vi "RTM Add Calculations.vi"(8 "error in (no error)":errorcluster, 11 "Node Ptr":u64 format="%.0x") -> (0 "error out":errorcluster)   [LabVIEW 2015, in "Waveform-Processing-Custom-Device System Explorer.lvlib"]
uses:
  Waveform-Processing-Custom-Device System Explorer.lvlib
  NationalInstruments.VeriStand.SystemStorageUI
  Classes/RunningAverageCalculation/RunningAverageCalculation.lvclass
  Classes/ScaledWaveformCalculation/ScaledWaveformCalculation.lvclass
  Classes/LatestValueCalculation/LatestValueCalculation.lvclass
  Shared/Constants.vi
  <vilib>/NI Veristand/Custom Device API/Get Item Property (String Array).vi
  NationalInstruments.VeriStand.SystemStorage
  Classes/WaveformCalculation/WaveformCalculation.lvclass
  <vilib>/NI VeriStand/Custom Device API/Custom Device API.lvlib
  <vilib>/NI VeriStand/UI Controls/System Definition Tree/NI_VS UI System Tree.lvlib
  Shared/Waveform-Processing-Custom-Device Shared.lvlib
  <vilib>/NI VeriStand/Custom Device Tools/Custom Device Utility Library/Custom Device Utility Library.lvlib
panel:
  in  "Select a calculation:":u16(ring)
  in  "OK Button":bool
  in  "TreeBrowserWF":refnum<k24>(container)
  in  "Tag":string
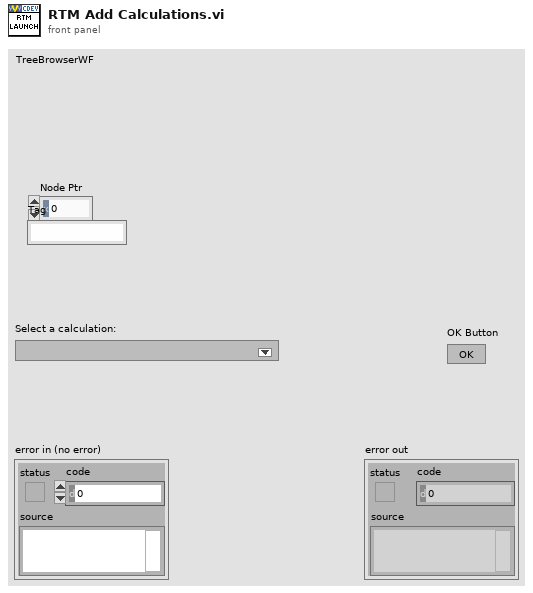
[diagram p1: front panel]
types:
  T1 = typedef "Custom Device API.lvlib/Custom Device Item Ref.ctl" = u64
  T2 = typedef "Custom Device API.lvlib/Custom Device Pointer.ctl" = refnum<k24>
  T3 = typedef "NI_VS UI System Tree.lvlib/Callback Type.ctl" = cluster{"Net Callbacks":refnum<k27>[], "Event":T4}
  T4 = typedef "NI_VS UI System Tree.lvlib/Net Event Data Ref.ctl" = refnum<user-event>
  T5 = typedef "NI_VS UI System Tree.lvlib/System Definition Tree Ref.ctl" = refnum<k24>
  T6 = typedef "Custom Device API.lvlib/Custom Device Item Info.ctl" = cluster{"Name":string, "Is Channel":bool, "GUID":string, "Is Waveform":bool}
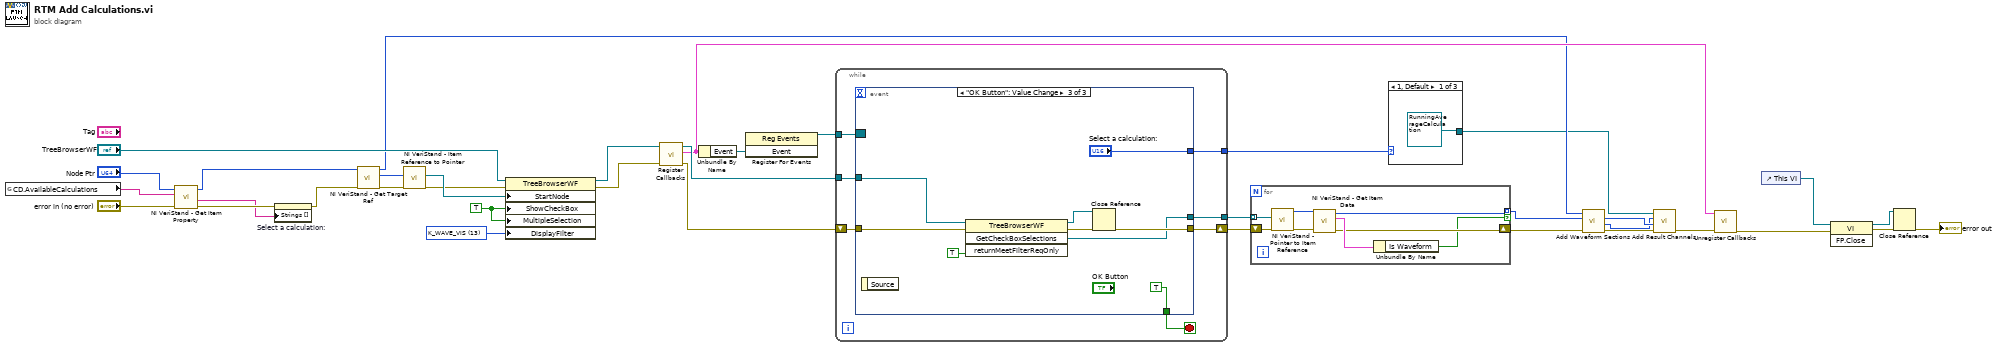
[diagram p0: block diagram]
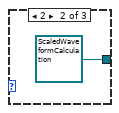
[diagram p2: hidden frame]
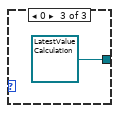
[diagram p3: hidden frame]
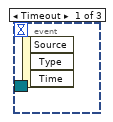
[diagram p4: hidden frame]
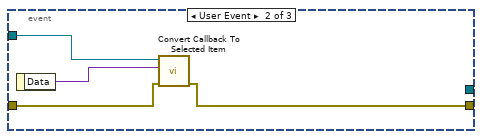
[diagram p5: hidden frame]
diagram:
  w24 = u8 13 items=["K_CHAN_R", "K_CHAN_W", "K_CHAN_RW", "K_CHAN_VOLT", "K_CHAN_FAULT", "K_ALL", "K_CUSTOM", "K_CHAN_R_VIS", "K_CHAN_W_VIS", "K_CHAN_RW_VIS", "K_CHAN_VOLT_VIS", "K_CHAN_FAULT_VIS", "K_WAVE", "K_WAVE_VIS", "K_WAVE_DBL", "K_WAVE_CDB", "K_WAVE_DBL_VIS", "K_WAVE_CDB_VIS"] ("filterType")
  w30 = TRUE ("ShowCheckBox")
  n1 = global read "Constants.vi" "CD.AvailableCalculations"() -> (w19:string)
  n2 = call-poly <vilib>:"NI VeriStand - Get Item Property.vi"("error in (no error)"="error in (no error)", "Property Name"=w19, "Item Ref in"="Node Ptr") -> ("error out"=w20:errorcluster, "Value"=w16:string[], "Item Ref out"=w12:T1)  [unwired: 5 in, 1 out]
  n3 = property on="Select a calculation:" class="Ring (strict)"(error in=w20, "Strings []"=w16) -> (error out=w13:errorcluster)  [unwired: 1 in, 1 out]
  n4 = call <vilib>:"NI VeriStand - Get Target Ref.vi"("error in"=w13, "Item Ref in"=w12) -> ("error out"=w14:errorcluster, "Target Ref"=w15:T1, "Item Ref out"=w10:T1)  [unwired: 6 in, 1 out]
  n5 = call <vilib>:"NI VeriStand - Item Reference to Pointer.vi"("error in (no error)"=w14, "Item Ref in"=w15) -> ("error out"=w22:errorcluster, "Node Pointer"=w33:T2)  [unwired: 6 in, 2 out]
  n6 = property class="TreeBrowserWF"(reference="TreeBrowserWF", error in=w22, "StartNode"=w33, "ShowCheckBox"=w30, "MultipleSelection"=w30, "DisplayFilter"=w24) -> (reference out=w31:refnum<k24>, error out=w32:errorcluster)
  n7 = call <vilib>:"Register Callbacks.vi"("error in (no error)"=w32, "System Definition Tree"=w31) -> ("error out"=w36:errorcluster, "Callbacks"=w21:T3, "System Definition Tree dup"=w35:T5)  [unwired: 7 in]
  n8 = Unbundle By Name(w21) -> ("Event"=w34:T4)
  n9 = register-events(w34) -> (reference out=w37:refnum<event-registration>)  [unwired: 2 in, 1 out]
  n10 = while {
    tunnel: w37 -> [w44]
    tunnel: w35 -> [w42]
    shift-right: [w41] -> w29
    shift-left: w36 -> [w43]
    tunnel: [w39] -> w6
    tunnel: [w38] -> w4
    stop <- w40 stop-if-true
    n11 = event shown="[2] \"OK Button\": Value Change" {
      selector: w44 -> [_ _ _]
      dyn-events: _ -> [_ _ _]
      timeout: _ -> [_ _ _]
      tunnel: w43 -> [_ w47 w55]
      tunnel: w42 -> [_ w46 w56]
      tunnel: [_ w45 w51] -> w41
      tunnel: [_ _ TRUE] -> w40
      tunnel: [_ _ "Select a calculation:"] -> w39
      tunnel: [_ _ w49] -> w38
      event Timeout {
        n12 = event-data() -> ()  [unwired: 1 in, 3 out]
      }
      event User Event {
        n13 = event-data() -> ("Data"=w48:variant)  [unwired: 1 in]
        n14 = call <vilib>:"Convert Callback To Selected Item.vi"("error in"=w47, "Data"=w48, "SystemDefinitionBrowser Ref"=w46) -> ("error out"=w45:errorcluster)  [unwired: 7 in, 1 out]
      }
      event "OK Button": Value Change {
        n15 = event-data() -> ()  [unwired: 1 in, 1 out]
        n16 = invoke class="TreeBrowserWF" method="GetCheckBoxSelections"(reference=w56, error in=w55, "returnMeetFilterReqOnly"=TRUE) -> (reference out=w52:T5, error out=w53:errorcluster, "GetCheckBoxSelections"=w49:refnum<k24>[])  [unwired: 1 in, 1 out]
        n17 = Close Reference(reference=w52, error in (no error)=w53) -> (error out=w51:errorcluster)
      }
    }
  }
  n18 = for {
    tunnel: w4 -> [w64] mode=indexing
    tunnel: [w61] -> w3 mode=indexing if=w58
    shift-right: [w59] -> w11
    shift-left: w29 -> [w65]
    n19 = call <vilib>:"NI VeriStand - Pointer to Item Reference.vi"("error in (no error)"=w65, "Node Pointer"=w64) -> ("error out"=w63:errorcluster, "Item Ref out"=w62:T1)  [unwired: 8 in]
    n20 = call <vilib>:"NI VeriStand - Get Item Data.vi"("error in (no error)"=w63, "Item Ref in"=w62) -> ("error out"=w59:errorcluster, "Item Info"=w60:T6, "Item Ref out"=w61:T1)  [unwired: 6 in, 1 out]
    n21 = Unbundle By Name(w60) -> ("Is Waveform"=w58:bool)
  }
  n22 = case shown="1, Default" w6 {
    tunnel: [refnum<class "RunningAverageCalculation.lvclass"> refnum ("RunningAverageCalculation.lvclass") refnum<class "ScaledWaveformCalculation.lvclass"> refnum ("ScaledWaveformCalculation.lvclass") refnum<class "LatestValueCalculation.lvclass"> refnum ("LatestValueCalculation.lvclass")] -> w5
    frame 1, Default {
    }
    frame 2 {
    }
    frame 0 {
    }
  }
  n23 = call "Add Waveform Sections.vi"("error in"=w11, "Source Waveform refs in"=w3, "CustomDevice Ref"=w10) -> ("error out"=w9:errorcluster, "Waveform Result Section refs"=w1:T1[], "Source Waveform refs out"=w2:T1[])  [unwired: 5 in, 1 out]
  n24 = call-dynamic "Add Result Channels.vi"("error in (no error)"=w9, "Selected Source Waveform items"=w2, "Selected Waveform Result Section Items"=w1, "WaveformCalculation in"=w5) -> ("error out"=w8:errorcluster)  [unwired: 6 in, 1 out]
  n25 = call <vilib>:"Unregister Callbacks.vi"("error in (no error)"=w8, "Callbacks"=w21) -> ("error out"=w7:errorcluster)  [unwired: 9 in]
  n26 = control-ref of="This VI"() -> (w28:refnum<vi>)
  n27 = invoke class="VI" method="FP.Close"(reference=w28, error in=w7) -> (reference out=w25:refnum<vi>, error out=w27:errorcluster)  [unwired: 1 in, 1 out]
  n28 = Close Reference(reference=w25, error in (no error)=w27) -> (error out=→"error out":errorcluster)
